vi "P&ID.vi"(6 "Valves":bool[](array[boolean]), 8 "Errors":bool[](array[boolean]), 9 "Warnings":bool[](array[boolean]), 10 "HasReadings":bool[](array[boolean]), 11 "Readings":dbl[](array[numeric])) -> ()   [LabVIEW 2018]
uses:
  3002b608-417b-4cc3-ad79-a17fc286b8bc.vi
panel:
  out "NC-OI":bool
  out "NC-FI":bool
  in  "Clear Errors":bool
  out "LC-E":dbl
  out "PT-3E":dbl
  out "PT-2E":dbl
  out "PT-1E":dbl
  out "FP-L":bool
  out "NC-FP":bool
  out "NC-OP":bool
  out "NC-O":bool
  out "NC-F":bool
  out "NO-P":bool
  out "NC-P":bool
  out "PT-CA":dbl
  out "PT-OA":dbl
  out "PT-FA":dbl
  out "FM-O":dbl
  out "FM-F":dbl
  out "TC-1F":dbl
  out "TC-2O":dbl
  out "TC-1O":dbl
  out "TC-3P":dbl
  out "TC-2P":dbl
  out "TC-1P":dbl
  out "PT-2O":dbl
  out "PT-1O":dbl
  out "PT-1F":dbl
  out "PT-L":dbl
  out "PT-3P":dbl
  out "PT-2P":dbl
  out "PT-1P":dbl
  # "Injector"
  # "NC-FI"
  # "NC-OI"
  # "Engine"
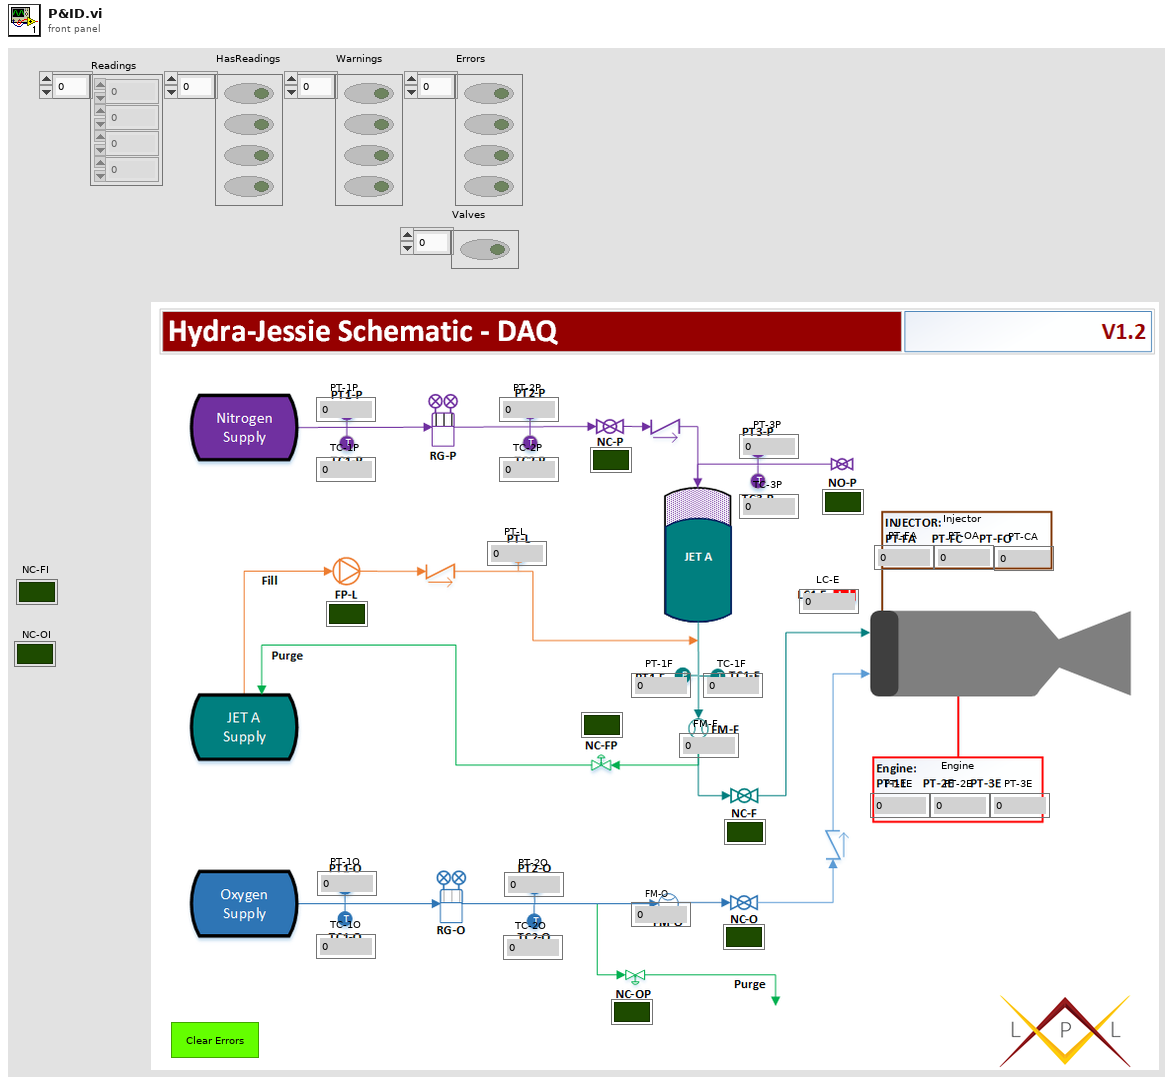
[diagram p1: front panel]
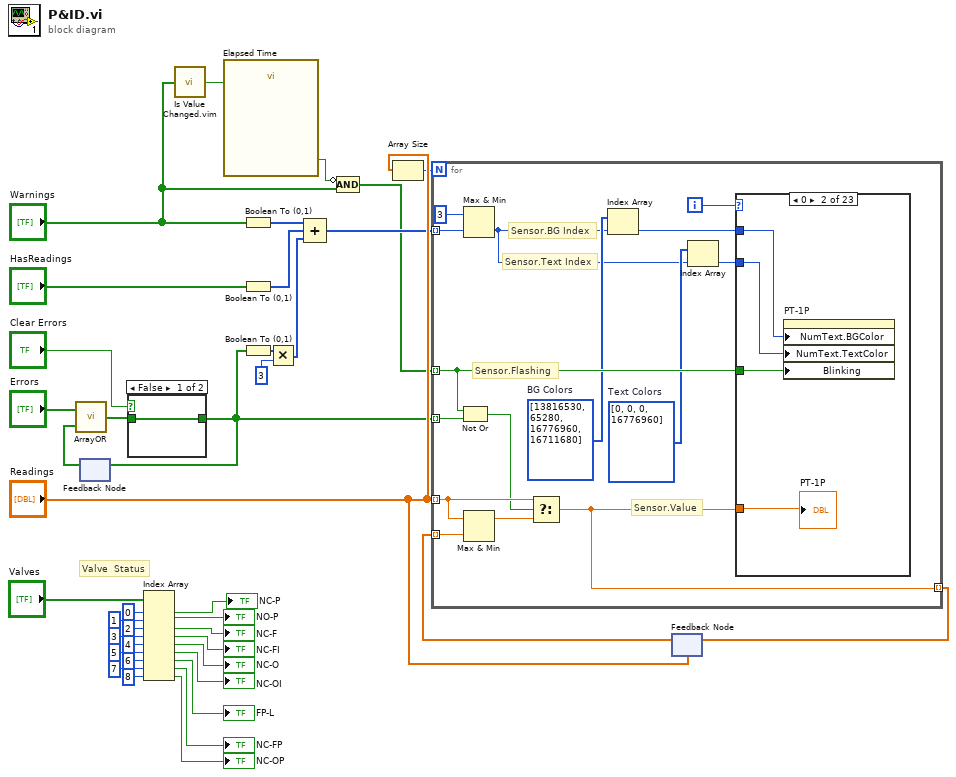
[diagram p0: block diagram]
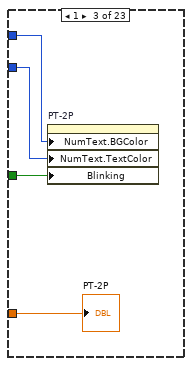
[diagram p3: hidden frame]
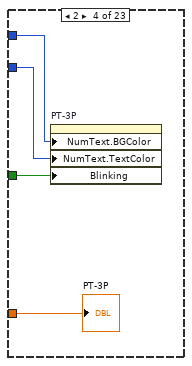
[diagram p4: hidden frame]
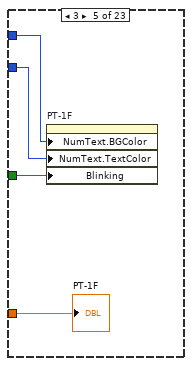
[diagram p5: hidden frame]
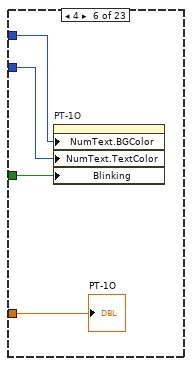
[diagram p6: hidden frame]
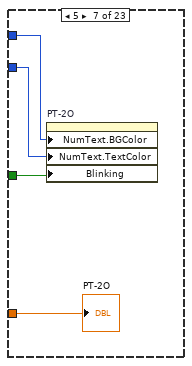
[diagram p7: hidden frame]
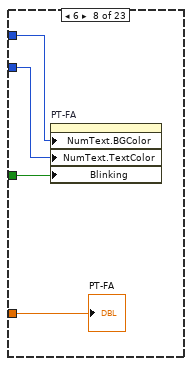
[diagram p8: hidden frame]
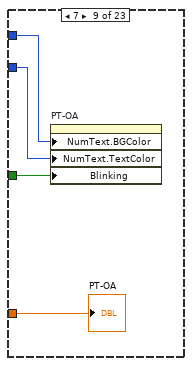
[diagram p9: hidden frame]
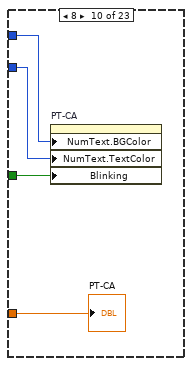
[diagram p10: hidden frame]
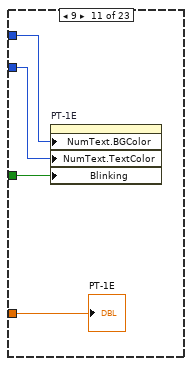
[diagram p11: hidden frame]
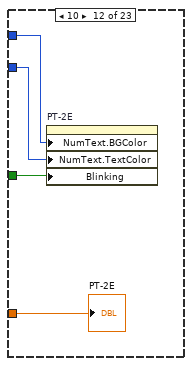
[diagram p12: hidden frame]
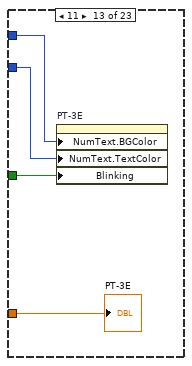
[diagram p13: hidden frame]
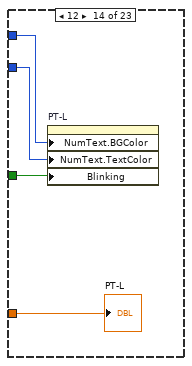
[diagram p14: hidden frame]
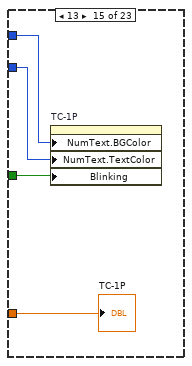
[diagram p15: hidden frame]
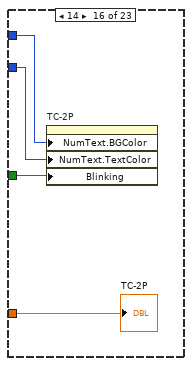
[diagram p16: hidden frame]
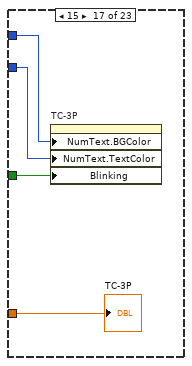
[diagram p17: hidden frame]
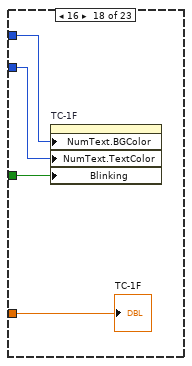
[diagram p18: hidden frame]
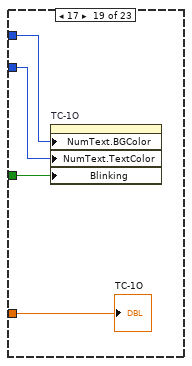
[diagram p19: hidden frame]
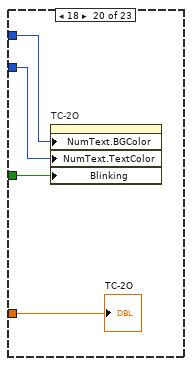
[diagram p20: hidden frame]
diagram:
  # "Valve  Status"
  n1 = feedback #1() -> (w7:bool[])  [unwired: 1 in]
  n2 = call "ArrayOR.vi"("Array 2"=w7, "Array 1"="Errors") -> ("1 || 2"=w9:bool[])
  n3 = case shown="False" "Clear Errors" {
    tunnel: [w40 w42] -> w13
    tunnel: w9 -> [w40 w43]
    frame False {
    }
    frame True {
      n4 = And(x=w43, y=FALSE) -> (x .and. y?=w42:bool[])
    }
  }
  n5 = feedback-in #1(w13) -> ()
  n6 = Index Array(array="Valves", index #1=0 ("index"), index #2=1 ("index"), index #3=2 ("index"), index #4=3 ("index"), index #5=4 ("index"), index #6=5 ("index"), index #7=6 ("index"), index #8=7 ("index"), index #9=8 ("index")) -> (element #1=→"NC-P":bool, element #2=→"NO-P":bool, element #3=→"NC-F":bool, element #4=→"NC-FI":bool, element #5=→"NC-O":bool, element #6=→"NC-OI":bool, element #7=→"FP-L":bool, element #8=→"NC-FP":bool, element #9=→"NC-OP":bool)
  n7 = call "Is Value Changed.vim"("value"="Warnings") -> ("changed or first call?"=w2:bool)
  n8 = call "Elapsed Time"("Reset"=w2) -> ("Time has Elapsed"=w33:bool)  [unwired: 11 in, 7 out]
  n9 = Boolean To (0,1)(Boolean="Warnings") -> (0, 1=w38:i16[])
  n10 = Boolean To (0,1)(Boolean="HasReadings") -> (0, 1=w37:i16[])
  n11 = Boolean To (0,1)(Boolean=w13) -> (0, 1=w36:i16[])
  n12 = Multiply(x=w36, y=i16 3) -> (x*y=w6:i16[])
  n13 = Compound Arithmetic op=ADD(w38, w37, w6) -> (w12:i16[])
  n14 = Compound Arithmetic op=AND(invert w33, "Warnings") -> (w11:bool[])
  n15 = Array Size(array="Readings") -> (size(s)=w10:i32)
  n16 = feedback #2("Readings") -> (w3:dbl[])
  n17 = for {
    N: w10 -> [_]
    tunnel: "Readings" -> [w57] mode=indexing
    tunnel: w13 -> [w55] mode=indexing
    tunnel: w11 -> [w53] mode=indexing
    tunnel: w12 -> [w45] mode=indexing
    tunnel: [w47] -> w4 mode=indexing
    tunnel: w3 -> [w46] mode=indexing
    i -> [w56]
    w49 = u32[] [0, 0, 0, 16776960]  # Text Colors
    w51 = u32[] [13816530, 65280, 16776960, 16711680]  # BG Colors
    # "Sensor.Value"
    # "Sensor.Text Index"
    # "Sensor.Flashing"
    # "Sensor.BG Index"
    n18 = Not Or(1:w55, 2:w53) -> (0:w54:bool)
    n19 = Max & Min(x=i16 3, y=w45) -> (min(x,y)=w44:i16)  [unwired: 1 out]
    n20 = Max & Min(x=w57, y=w46) -> (max(x,y)=w58:dbl)  [unwired: 1 out]
    n21 = Select(t=w57, s=w54, f=w58) -> (s? t:f=w47:dbl)
    n22 = Index Array(array=w51, index=w44) -> (element=w52:u32)
    n23 = Index Array(array=w49, index=w44) -> (element=w50:u32)
    n24 = case shown="0" w56 {
      tunnel: w50 -> [_ w61 w63 w68 w72 w76 w80 w83 w87 w91 w95 w100 w104 w108 w111 w115 w119 w123 w127 w131 w135 w139 w143]
      tunnel: w52 -> [_ w60 w64 w69 w73 w77 w81 w84 w88 w92 w96 w101 w105 w109 w112 w116 w120 w124 w128 w132 w136 w140 w144]
      tunnel: w53 -> [_ w62 w65 w67 w71 w75 w79 w85 w89 w93 w97 w99 w103 w107 w113 w117 w121 w125 w129 w133 w137 w141 w145]
      tunnel: w47 -> [_ w59 w66 w70 w74 w78 w82 w86 w90 w94 w98 w102 w106 w110 w114 w118 w122 w126 w130 w134 w138 w142 w146]
      frame Default {
      }
      frame 0 {
        n25 = property on="PT-1P" class="DigNum (strict)"("NumText.BGColor"=w60, "NumText.TextColor"=w61, "Blinking"=w62) -> ()  [unwired: 2 in, 2 out]
        "PT-1P" <- w59
      }
      frame 1 {
        n26 = property on="PT-2P" class="DigNum (strict)"("NumText.BGColor"=w64, "NumText.TextColor"=w63, "Blinking"=w65) -> ()  [unwired: 2 in, 2 out]
        "PT-2P" <- w66
      }
      frame 2 {
        n27 = property on="PT-3P" class="DigNum (strict)"("NumText.BGColor"=w69, "NumText.TextColor"=w68, "Blinking"=w67) -> ()  [unwired: 2 in, 2 out]
        "PT-3P" <- w70
      }
      frame 3 {
        n28 = property on="PT-1F" class="DigNum (strict)"("NumText.BGColor"=w73, "NumText.TextColor"=w72, "Blinking"=w71) -> ()  [unwired: 2 in, 2 out]
        "PT-1F" <- w74
      }
      frame 4 {
        n29 = property on="PT-1O" class="DigNum (strict)"("NumText.BGColor"=w77, "NumText.TextColor"=w76, "Blinking"=w75) -> ()  [unwired: 2 in, 2 out]
        "PT-1O" <- w78
      }
      frame 5 {
        n30 = property on="PT-2O" class="DigNum (strict)"("NumText.BGColor"=w81, "NumText.TextColor"=w80, "Blinking"=w79) -> ()  [unwired: 2 in, 2 out]
        "PT-2O" <- w82
      }
      frame 6 {
        n31 = property on="PT-FA" class="DigNum (strict)"("NumText.BGColor"=w84, "NumText.TextColor"=w83, "Blinking"=w85) -> ()  [unwired: 2 in, 2 out]
        "PT-FA" <- w86
      }
      frame 7 {
        n32 = property on="PT-OA" class="DigNum (strict)"("NumText.BGColor"=w88, "NumText.TextColor"=w87, "Blinking"=w89) -> ()  [unwired: 2 in, 2 out]
        "PT-OA" <- w90
      }
      frame 8 {
        n33 = property on="PT-CA" class="DigNum (strict)"("NumText.BGColor"=w92, "NumText.TextColor"=w91, "Blinking"=w93) -> ()  [unwired: 2 in, 2 out]
        "PT-CA" <- w94
      }
      frame 9 {
        n34 = property on="PT-1E" class="DigNum (strict)"("NumText.BGColor"=w96, "NumText.TextColor"=w95, "Blinking"=w97) -> ()  [unwired: 2 in, 2 out]
        "PT-1E" <- w98
      }
      frame 10 {
        n35 = property on="PT-2E" class="DigNum (strict)"("NumText.BGColor"=w101, "NumText.TextColor"=w100, "Blinking"=w99) -> ()  [unwired: 2 in, 2 out]
        "PT-2E" <- w102
      }
      frame 11 {
        n36 = property on="PT-3E" class="DigNum (strict)"("NumText.BGColor"=w105, "NumText.TextColor"=w104, "Blinking"=w103) -> ()  [unwired: 2 in, 2 out]
        "PT-3E" <- w106
      }
      frame 12 {
        n37 = property on="PT-L" class="DigNum (strict)"("NumText.BGColor"=w109, "NumText.TextColor"=w108, "Blinking"=w107) -> ()  [unwired: 2 in, 2 out]
        "PT-L" <- w110
      }
      frame 13 {
        n38 = property on="TC-1P" class="DigNum (strict)"("NumText.BGColor"=w112, "NumText.TextColor"=w111, "Blinking"=w113) -> ()  [unwired: 2 in, 2 out]
        "TC-1P" <- w114
      }
      frame 14 {
        n39 = property on="TC-2P" class="DigNum (strict)"("NumText.BGColor"=w116, "NumText.TextColor"=w115, "Blinking"=w117) -> ()  [unwired: 2 in, 2 out]
        "TC-2P" <- w118
      }
      frame 15 {
        n40 = property on="TC-3P" class="DigNum (strict)"("NumText.BGColor"=w120, "NumText.TextColor"=w119, "Blinking"=w121) -> ()  [unwired: 2 in, 2 out]
        "TC-3P" <- w122
      }
      frame 16 {
        n41 = property on="TC-1F" class="DigNum (strict)"("NumText.BGColor"=w124, "NumText.TextColor"=w123, "Blinking"=w125) -> ()  [unwired: 2 in, 2 out]
        "TC-1F" <- w126
      }
      frame 17 {
        n42 = property on="TC-1O" class="DigNum (strict)"("NumText.BGColor"=w128, "NumText.TextColor"=w127, "Blinking"=w129) -> ()  [unwired: 2 in, 2 out]
        "TC-1O" <- w130
      }
      frame 18 {
        n43 = property on="TC-2O" class="DigNum (strict)"("NumText.BGColor"=w132, "NumText.TextColor"=w131, "Blinking"=w133) -> ()  [unwired: 2 in, 2 out]
        "TC-2O" <- w134
      }
      frame 19 {
        n44 = property on="FM-F" class="DigNum (strict)"("NumText.BGColor"=w136, "NumText.TextColor"=w135, "Blinking"=w137) -> ()  [unwired: 2 in, 2 out]
        "FM-F" <- w138
      }
      frame 20 {
        n45 = property on="FM-O" class="DigNum (strict)"("NumText.BGColor"=w140, "NumText.TextColor"=w139, "Blinking"=w141) -> ()  [unwired: 2 in, 2 out]
        "FM-O" <- w142
      }
      frame 21 {
        n46 = property on="LC-E" class="DigNum (strict)"("NumText.BGColor"=w144, "NumText.TextColor"=w143, "Blinking"=w145) -> ()  [unwired: 2 in, 2 out]
        "LC-E" <- w146
      }
    }
  }
  n47 = feedback-in #2(w4) -> ()
